vi "Global 1.vi"() -> ()   [LabVIEW 2012]
panel:
  in  "stop":bool
  out "Phase":string
  out "Frequency":string
  out "VR":string
  out "VY":string
  out "VX":string
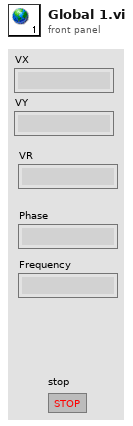
[diagram p1: front panel]
diagram:
